vi "Temperature Monitor (Demo).vi"() -> ()   [LabVIEW 2014]
doc: "This VI is the solution to an exercise in the LabVIEW Core I course.\n\nIt is used to demonstrate While loops and waveform charts. This VI simulates a temperature reading once every 500 ms and plots the data in a strip chart."
panel:
  out "Temperature History":dbl(graph)
  in  "Power":bool=TRUE
  # "ON\n\nOFF"
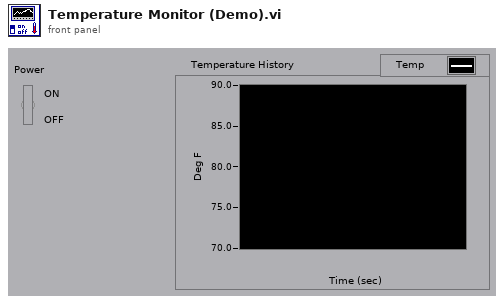
[diagram p1: front panel]
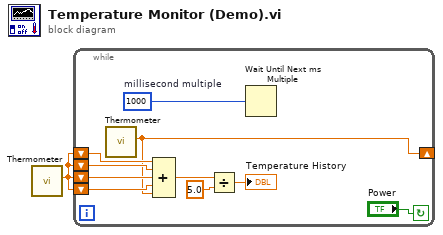
[diagram p0: block diagram]
diagram:
  n1 = call "Thermometer.vi"() -> ("Temperature"=w1:dbl)  [unwired: 10 in, 1 out]
  n2 = while {
    shift-right: [w2] -> _
    shift-left: w1 -> [w6]
    shift-left: w1 -> [w5]
    shift-left: w1 -> [w4]
    shift-left: w1 -> [w3]
    stop <- "Power" continue-if-true
    w10 = u32 1000  # millisecond multiple
    n3 = call "Thermometer.vi"() -> ("Temperature"=w2:dbl)  [unwired: 10 in, 1 out]
    n4 = Compound Arithmetic op=ADD(w6, w5, w4, w3, w2) -> (w7:dbl)
    n5 = Divide(x=w7, y=5.0) -> (x/y=→"Temperature History":dbl)
    n6 = Wait Until Next ms Multiple(millisecond multiple=w10) -> ()  [unwired: 1 out]
  }
